vi "Chirp.vi"(0 "Pulser":T1, 1 "Agilent In":refnum<visa-resource-name>="GPIB::10::INSTR", 2 "Tabor In":refnum<k15>="Tabor2182", 3 "error in (no error)":errorcluster, 4 "Use Address?":bool=TRUE) -> (6 "error out":errorcluster)   [LabVIEW 2022 SP3]
uses:
  Pulsers/pulser.ctl
  <vilib>/Analysis/NI_AALPro.lvlib
  <vilib>/Analysis/NI_AALBase.lvlib
  Motion Controllers/-MotionRoutines/MotionGlobals.vi
  Pulsers/PulserGlobals.vi
  <vilib>/Utility/file.llb/Read From Spreadsheet File (DBL).vi
panel:
  in  "resource name":refnum<k15>
  in  "Vpp":dbl=0.105 min=0.05 max=1.0 format="%.2f"
  in  "duration tone (us)":sgl=4.0
  in  "fb (MHz)":dbl=10.0 format="%0.2f"
  in  "Tabor mode":enum32{"Arb Wave", "Sequence"}(tab)
  in  "Upload Wave?":bool
  out "Waveform Handles":i32[](array[numeric])
  in  "Clear Arb":bool
  in  "Arb Mode":bool
  in  "Arb Seg":i32=1 min=1
  in  "Scaling fac":dbl=1.0 min=-1.0 max=1.0 format="%.2f"
  in  "Clear Seq Tab":bool
  in  "Sequence Table":i32[][](array[numeric])=[[1, 1], [2, 1]] caption="Seg#      Rpt#"
  in  "Upload Seq Tab":bool
  out "seq handle":i32
  in  "dead time (us)":sgl=100.0
  in  "Tukey":dbl=0.15
  in  "Lobe ratio":dbl=90.0
  in  "duration chirp (us)":sgl=4.0
  in  "f2 (MHz)":dbl=80.0 format="%0.2f"
  in  "f1 (MHz)":dbl=10.0 format="%0.2f"
  out "Pts in Waveform":i32
  in  "Chirp File":path=path "F:/Temp/Chirp Test/Chirp12to68MHz_Tabor_9p_4us.txt"
  in  "Data Source":T2(ring)=enum."Calculate Chirp"
  in  "Func Gen":enum32{"Tabor1281", "Tabor2182", "Agilent"}(tab)=enum."Tabor2182"
  in  "T1281 D/A Rate (MHz)":dbl=1150.0 min=1.0 max=1190.0
  in  "T2182 D/A Rate (MHz)":dbl=2300.0 min=1.0 max=2300.0
  in  "User Def. Wfm Name":string="ARB_1"
  in  "samples":i32=16384
  in  "stop":bool
  out "Catalog":string
  out "Free Memory Slots":i32
  out "FFT":T3(graph)
  out "waveform":cluster{i32, dbl, dbl[]}(graph)
  # "f1 can be greater than f2. Make Tukey negative to invert chirp.\n\nUse fb for Burst and Monocycle.\n\nDuration for Chirp and Burst.\nDead time for ARFI Burst"
  # "Download before 1 Vpp change"
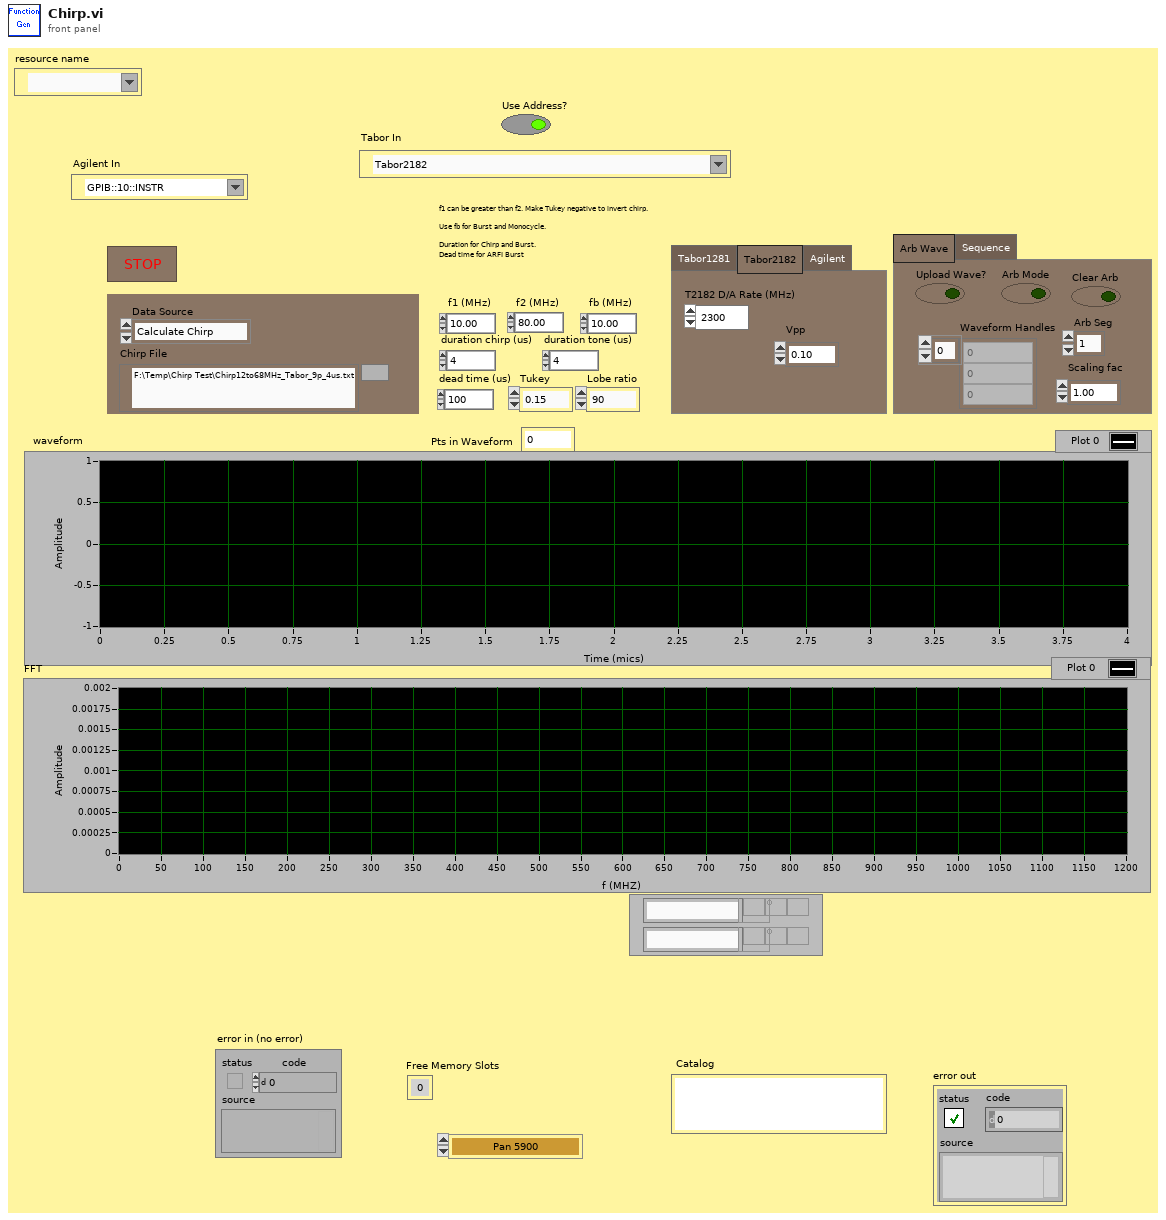
[diagram p1: front panel]
types:
  T1 = typedef "pulser.ctl" = enum16{"Pan 5900", "Daxsonics", "Agilent 33xxx", "UTEX", "JSR", "WMC Mono-Cycle", "No Pulser", "NYU AVTECH", "Tabor W1281A", "Pan 5800", "Unlisted", "Tabor WX2182B"}
  T2 = enum16{"Load Text File", "Calculate Chirp", "MonoCycle", "ToneBurst", "ARFI Burst", "ARFI Burst w/ Chirp"}
  T3 = cluster{i32, "df":dbl, "Power Spectrum (V^2 rms)":dbl[]}
  T4 = cluster{"instrument handle out":refnum<k15>, "instrument handle out":refnum<k15>, "Agilent In":refnum<visa-resource-name>}
  T5 = cluster{"Therapy frequency (MHz)":dbl, "Therapy amplitude (mV)":dbl, "time therapy on (s)":dbl, "Therapy Delay (ms) ":dbl, "Time (s)":dbl}
  T6 = cluster{"f1 (MHz)":dbl, "f2 (MHz)":dbl, "Tukey":dbl, "duration chirp (us)":sgl}
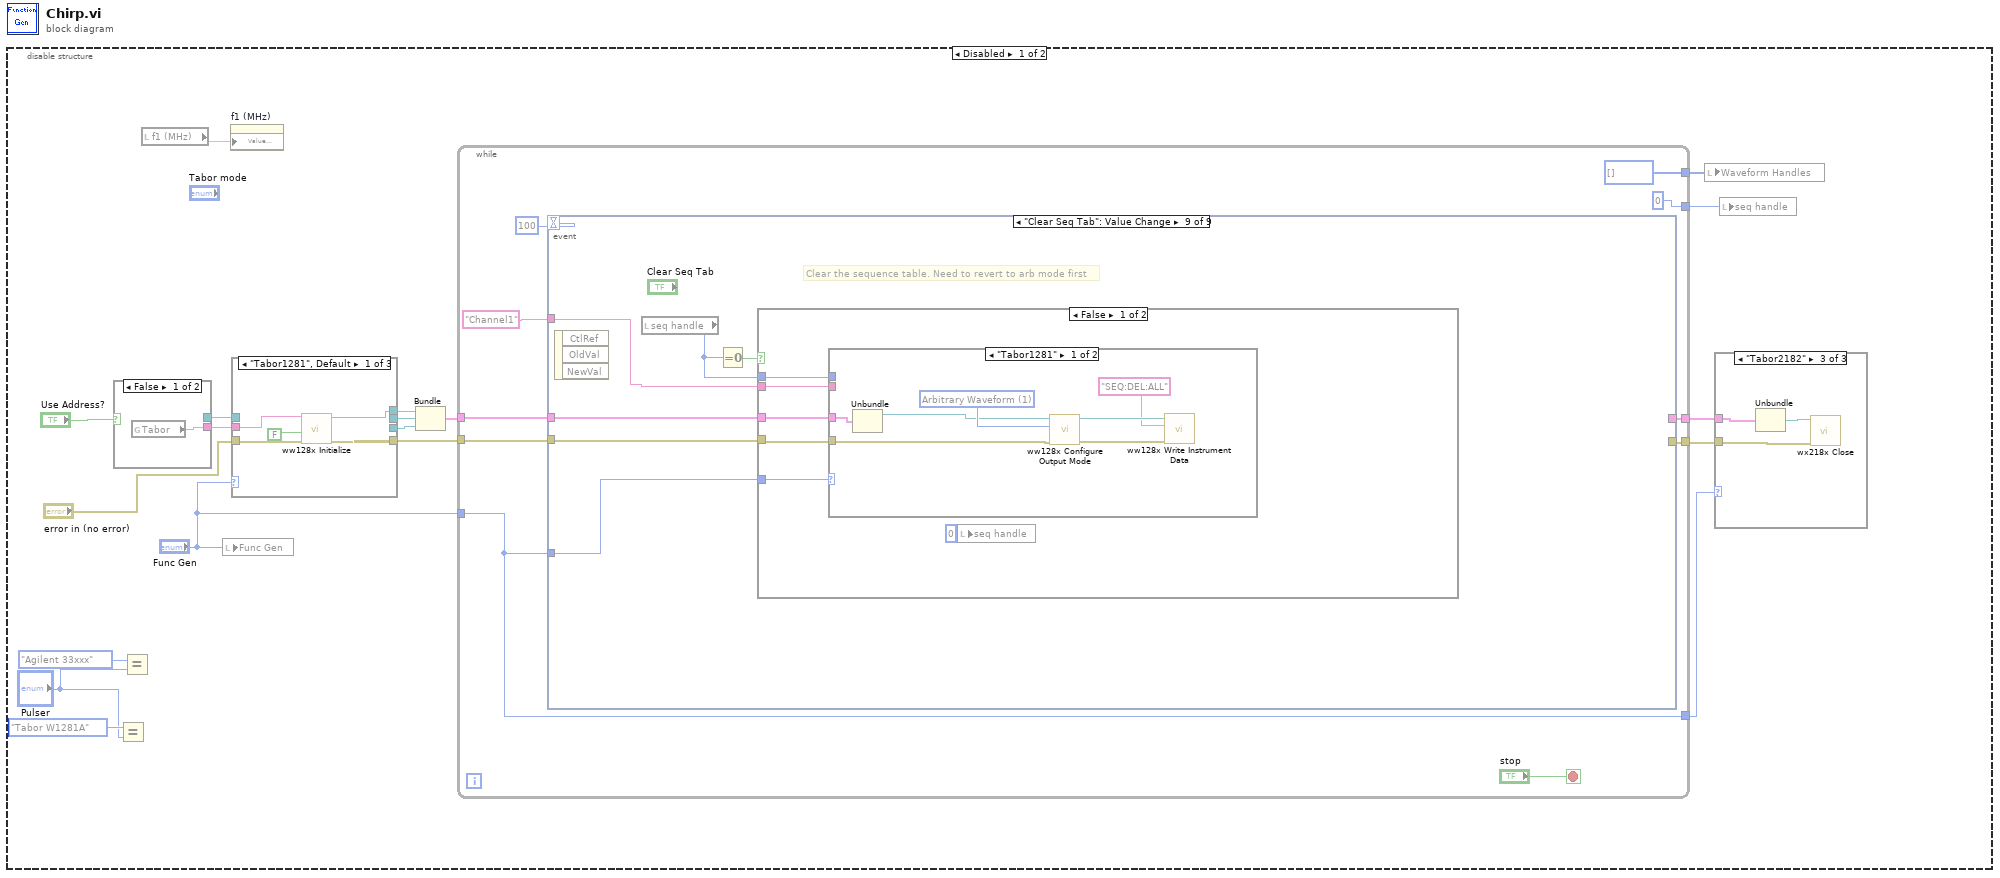
[diagram p0: block diagram]
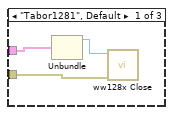
[diagram p2: hidden frame]
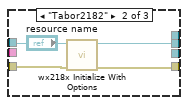
[diagram p4: hidden frame]
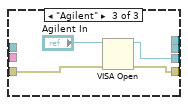
[diagram p5: hidden frame]
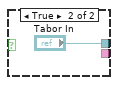
[diagram p6: hidden frame]
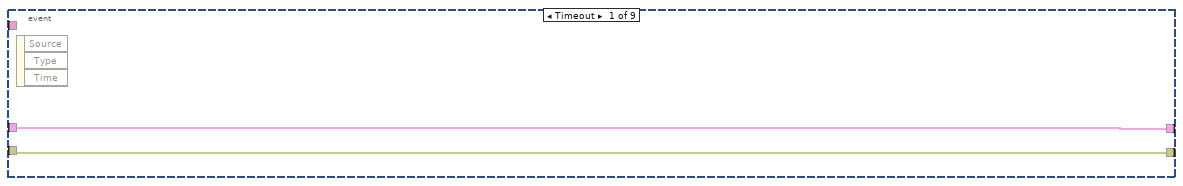
[diagram p7: hidden frame]
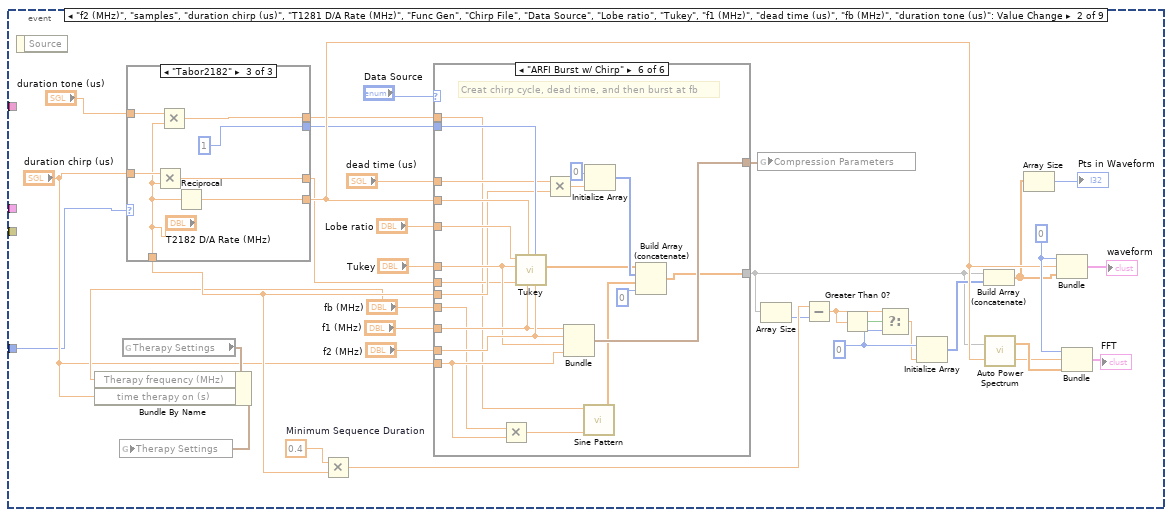
[diagram p8: hidden frame]
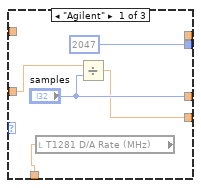
[diagram p9: hidden frame]
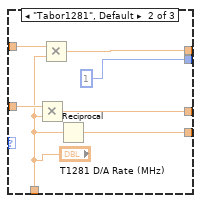
[diagram p10: hidden frame]
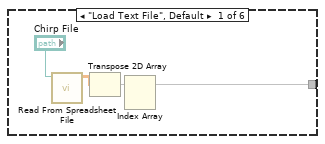
[diagram p11: hidden frame]
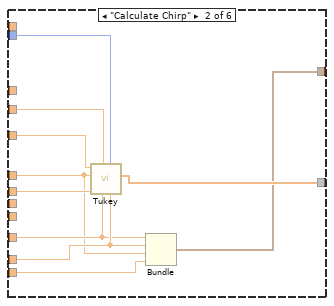
[diagram p12: hidden frame]
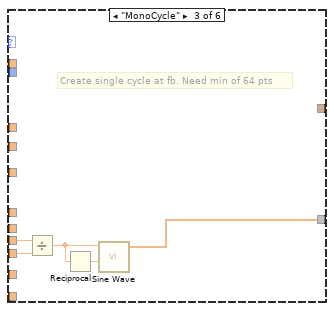
[diagram p13: hidden frame]
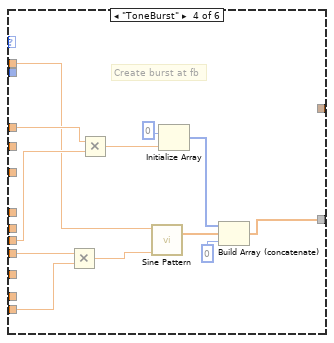
[diagram p14: hidden frame]
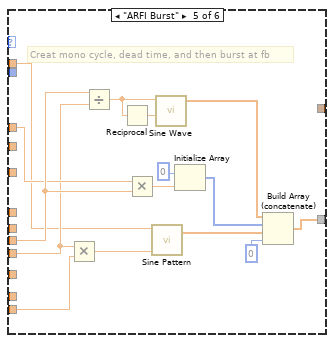
[diagram p15: hidden frame]
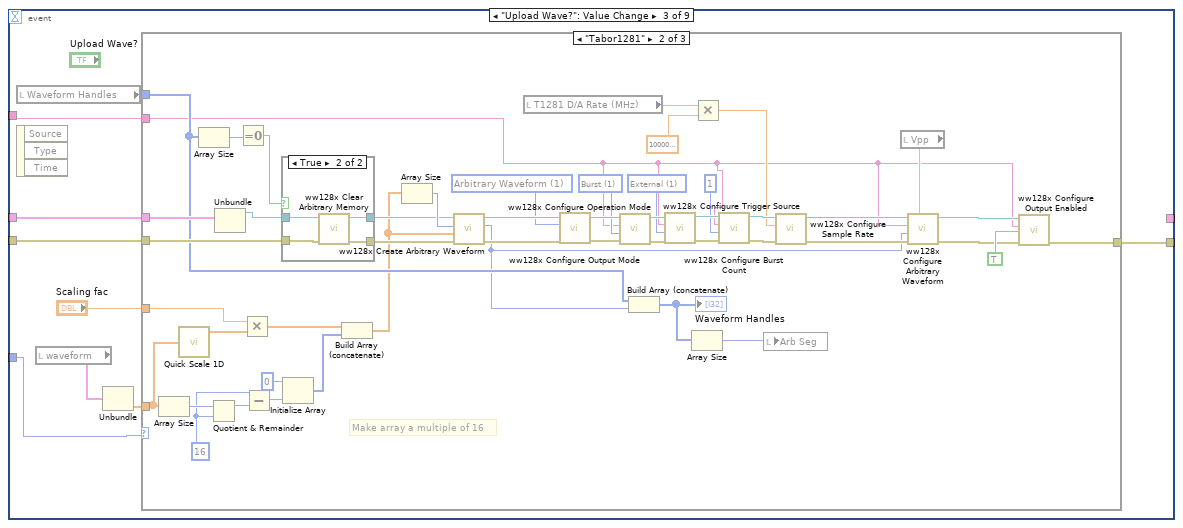
[diagram p16: hidden frame]
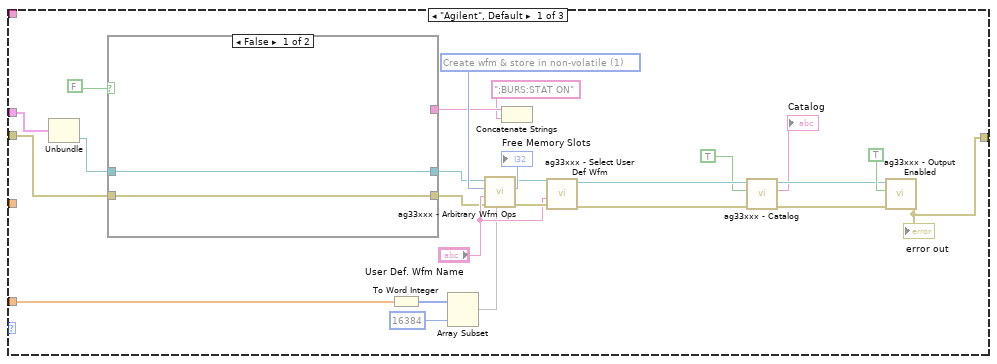
[diagram p17: hidden frame]
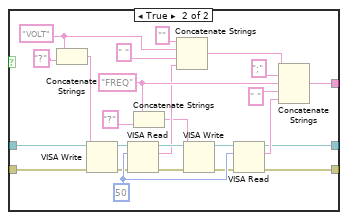
[diagram p18: hidden frame]
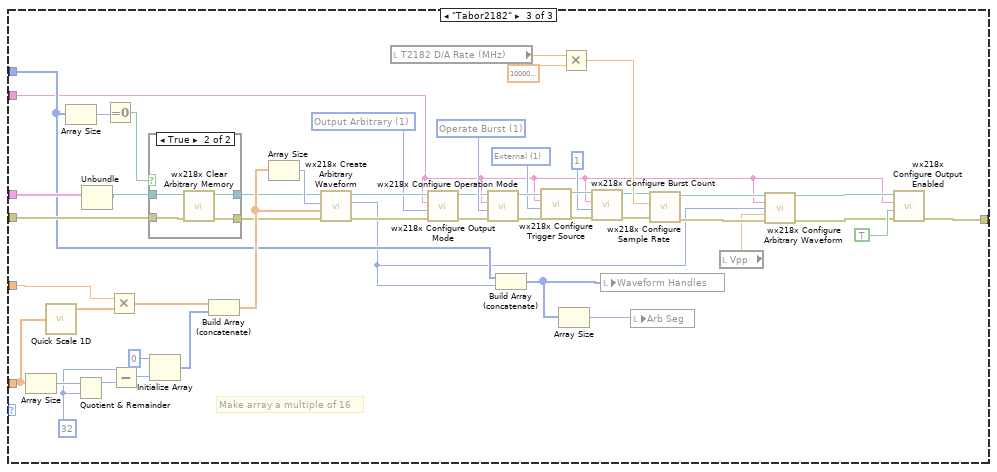
[diagram p20: hidden frame]
diagram:
  n1 = disable-structure shown="Disabled" {
    frame Disabled {
      n2 = case shown="False" "Use Address?" {
        tunnel: [w39 _] -> w2
        tunnel: [_ "Tabor In"] -> w1
        frame False {
          n3 = global read "PulserGlobals.vi" "Tabor"() -> (w39:string)
        }
        frame True {
        }
      }
      n4 = Equal?(x=pulser."Tabor W1281A", y="Pulser") -> ()  [unwired: 1 out]
      n5 = Equal?(x=pulser."Agilent 33xxx", y="Pulser") -> ()  [unwired: 1 out]
      n6 = local read "f1 (MHz)"() -> (w19:dbl)
      n7 = local write "Func Gen"("Func Gen") -> ()
      n8 = property on="f1 (MHz)" class="DigNum (strict)"("Value (Signaling)"=w19) -> ()  [unwired: 2 in, 2 out]
      n9 = case shown="\"Tabor1281\", Default" "Func Gen" {
        tunnel: [w29 w33 w36] -> w16
        tunnel: w1 -> [_ w31 _]
        tunnel: [w28 _ _] -> w12
        tunnel: [_ w34 _] -> w11
        tunnel: [_ _ w37] -> w7
        tunnel: "error in (no error)" -> [w27 w32 w35]
        tunnel: w2 -> [w26 _ _]
        frame "Tabor1281", Default {
          n10 = call <instrlib>:"ww128x Initialize.vi"("error in (no error)"=w27, "reset device (Yes)"=FALSE ("reset device"), "resource name"=w26) -> ("error out"=w29:errorcluster, "instrument handle out"=w28:refnum<k15>)  [unwired: 1 in, 6 out]
        }
        frame "Tabor2182" {
          n11 = call <instrlib>:"wx218x Initialize With Options.vi"("error in (no error)"=w32, "resource name"=w31) -> ("error out"=w33:errorcluster, "instrument handle out"=w34:refnum<k15>)  [unwired: 8 in]
        }
        frame "Agilent" {
          n12 = VISA Open(error in (no error)=w35, VISA resource name="Agilent In") -> (VISA resource name=w37:refnum<visa-resource-name>, error out=w36:errorcluster)  [unwired: 3 in]
        }
      }
      n13 = Bundle("instrument handle out"=w12, "instrument handle out"=w11, "Agilent In"=w7) -> (w10:T4)  [unwired: 1 in]
      n14 = while {
        tunnel: [w48] -> w18
        tunnel: [w47] -> w17
        tunnel: w10 -> [w46]
        tunnel: w16 -> [w45]
        tunnel: [i32[] [] ("Waveform Handles")] -> w15
        tunnel: [0 ("seq handle")] -> w13
        tunnel: "Func Gen" -> [w41]
        tunnel: [w41] -> w9
        stop <- "stop" stop-if-true
        n15 = event shown="[8] \"Clear Seq Tab\": Value Change" {
          selector: _ -> [_ _ _ _ _ _ _ _ _]
          dyn-events: _ -> [_ _ _ _ _ _ _ _ _]
          timeout: 100 -> [_ _ _ _ _ _ _ _ _]
          tunnel: [w52 _ _ _ _ _ _ _ _] -> w48
          tunnel: [w51 _ w173 _ w387 _ _ _ _] -> w47
          tunnel: w46 -> [w52 _ w179 w344 w393 w415 w469 w482 w513]
          tunnel: w45 -> [w51 _ w178 w348 w395 w416 w470 w486 w515]
          tunnel: "Channel1" -> [_ _ w175 w342 w392 w414 w467 w480 w510]
          tunnel: w41 -> [_ w53 w174 w343 w388 w413 w468 w481 w511]
          event Timeout {
            n16 = event-data() -> ()  [unwired: 4 out]
          }
          event "f2 (MHz)", "samples", "duration chirp (us)", "T1281 D/A Rate (MHz)", "Func Gen", "Chirp File", "Data Source", "Lobe ratio", "Tukey", "f1 (MHz)", "dead time (us)", "fb (MHz)", "duration tone (us)": Value Change {
            w65 = 0.4  # Minimum Sequence Duration
            w71 = 0
            w83 = 0
            n17 = event-data() -> ()  [unwired: 2 out]
            n18 = global read "PulserGlobals.vi" "Therapy Settings"() -> (w57:T5)
            n19 = Bundle By Name(cluster=w57, "Therapy frequency (MHz)"="fb (MHz)", "time therapy on (s)"="duration chirp (us)") -> (w56:T5)
            n20 = global write "PulserGlobals.vi" "Therapy Settings"(w56) -> ()
            n21 = case shown="\"Tabor2182\"" w53 {
              tunnel: ["samples" w97 w104] -> w78
              tunnel: "duration chirp (us)" -> [w91 w98 w105]
              tunnel: [w87 "T1281 D/A Rate (MHz)" "T2182 D/A Rate (MHz)"] -> w66
              tunnel: [w89 w96 w103] -> w79
              tunnel: [2047 1 1] -> w75
              tunnel: "duration tone (us)" -> [_ w94 w101]
              tunnel: [_ w93 w100] -> w58
              frame "Agilent" {
                n22 = local read "T1281 D/A Rate (MHz)"() -> (w87:dbl)
                n23 = Divide(x=w91, y="samples") -> (x/y=w89:sgl)
              }
              frame "Tabor1281", Default {
                n24 = Multiply(x=w98, y="T1281 D/A Rate (MHz)") -> (x*y=w97:dbl)
                n25 = Multiply(x=w94, y="T1281 D/A Rate (MHz)") -> (x*y=w93:dbl)
                n26 = Reciprocal(x="T1281 D/A Rate (MHz)") -> (1/x=w96:dbl)
              }
              frame "Tabor2182" {
                n27 = Multiply(x=w105, y="T2182 D/A Rate (MHz)") -> (x*y=w104:dbl)
                n28 = Multiply(x=w101, y="T2182 D/A Rate (MHz)") -> (x*y=w100:dbl)
                n29 = Reciprocal(x="T2182 D/A Rate (MHz)") -> (1/x=w103:dbl)
              }
            }
            n30 = Multiply(x=w65, y=w66) -> (x*y=w64:dbl)
            n31 = case shown="\"ARFI Burst w/ Chirp\"" "Data Source" {
              tunnel: [w107 w119 w121 w132 w147 w156] -> w67
              tunnel: "f1 (MHz)" -> [_ w115 _ _ _ w170]
              tunnel: "f2 (MHz)" -> [_ w116 _ _ _ w171]
              tunnel: w79 -> [_ w118 _ _ _ w172]
              tunnel: w78 -> [_ w117 _ _ _ w157]
              tunnel: "Lobe ratio" -> [_ w114 _ _ _ w169]
              tunnel: "Tukey" -> [_ w113 _ _ _ w168]
              tunnel: "duration chirp (us)" -> [_ w112 _ w135 w150 w154]
              tunnel: w75 -> [_ w111 _ _ _ w167]
              tunnel: w66 -> [_ _ w122 w127 w140 w158]
              tunnel: [_ w110 _ _ _ w166] -> w61
              tunnel: "dead time (us)" -> [_ _ _ w129 w139 w159]
              tunnel: "fb (MHz)" -> [_ _ w120 w126 w138 w153]
              tunnel: w58 -> [_ _ _ w125 w137 w152]
              frame "Load Text File", Default {
                n32 = call-poly <vilib>:"Read From Spreadsheet File.vi"("file path (dialog if empty)"="Chirp File") -> ("all rows"=w108:dbl[][])  [unwired: 3 in, 7 out]
                n33 = Transpose 2D Array(2D array=w108) -> (transposed array=w106:dbl[][])
                n34 = Index Array(array=w106) -> (element=w107:dbl[])  [unwired: 2 in]
              }
              frame "Calculate Chirp" {
                n35 = call "Tukey.vi"("f2 (MHz)"=w116, "Pk Value"=w111, "f1 (MHz)"=w115, "Samp Rate (mics)"=w118, "Pts"=w117, "Tukey"=w113, "Lobe ratio"=w114) -> ("Tukey Chirp"=w119:dbl[])  [unwired: 4 out]
                n36 = Bundle("f1 (MHz)"=w115, "f2 (MHz)"=w116, "Tukey"=w113, "duration chirp (us)"=w112) -> (w110:T6)  [unwired: 1 out]
              }
              frame "MonoCycle" {
                # "Create single cycle at fb. Need min of 64 pts"
                n37 = Divide(x=w122, y=w120) -> (x/y=w124:dbl)
                n38 = Reciprocal(x=w124) -> (1/x=w123:dbl)
                n39 = call <vilib>:"Sine Wave.vi"("samples"=w124, "frequency"=w123) -> ("sine wave"=w121:dbl[])  [unwired: 3 in, 2 out]
              }
              frame "ToneBurst" {
                # "Create burst at fb"
                n40 = Multiply(x=w126, y=w135) -> (x*y=w136:dbl)
                n41 = Multiply(x=w129, y=w127) -> (x*y=w130:dbl)
                n42 = call <vilib>:"Sine Pattern.vi"("cycles"=w136, "samples"=w125) -> ("Sinusoidal Pattern"=w134:dbl[])  [unwired: 2 in, 1 out]
                n43 = Initialize Array(0, w130) -> (w128:i32[])
                n44 = Build Array (concatenate)(w128, w134, 0) -> (w132:dbl[])
              }
              frame "ARFI Burst" {
                # "Creat mono cycle, dead time, and then burst at fb"
                n45 = Multiply(x=w138, y=w150) -> (x*y=w151:dbl)
                n46 = Divide(x=w140, y=w138) -> (x/y=w146:dbl)
                n47 = Reciprocal(x=w146) -> (1/x=w145:dbl)
                n48 = Multiply(x=w139, y=w140) -> (x*y=w143:dbl)
                n49 = call <vilib>:"Sine Pattern.vi"("cycles"=w151, "samples"=w137) -> ("Sinusoidal Pattern"=w149:dbl[])  [unwired: 2 in, 1 out]
                n50 = call <vilib>:"Sine Wave.vi"("samples"=w146, "frequency"=w145) -> ("sine wave"=w142:dbl[])  [unwired: 3 in, 2 out]
                n51 = Initialize Array(0, w143) -> (w141:i32[])
                n52 = Build Array (concatenate)(w142, w141, w149, 0) -> (w147:dbl[])
              }
              frame "ARFI Burst w/ Chirp" {
                # "Creat chirp cycle, dead time, and then burst at fb"
                n53 = Multiply(x=w153, y=w154) -> (x*y=w165:dbl)
                n54 = call "Tukey.vi"("f2 (MHz)"=w171, "Pk Value"=w167, "f1 (MHz)"=w170, "Samp Rate (mics)"=w172, "Pts"=w157, "Tukey"=w168, "Lobe ratio"=w169) -> ("Tukey Chirp"=w155:dbl[])  [unwired: 4 out]
                n55 = Multiply(x=w159, y=w158) -> (x*y=w161:dbl)
                n56 = Bundle("f1 (MHz)"=w170, "f2 (MHz)"=w171, "Tukey"=w168, "duration chirp (us)"=w154) -> (w166:T6)  [unwired: 1 out]
                n57 = call <vilib>:"Sine Pattern.vi"("cycles"=w165, "samples"=w152) -> ("Sinusoidal Pattern"=w164:dbl[])  [unwired: 2 in, 1 out]
                n58 = Initialize Array(0, w161) -> (w160:i32[])
                n59 = Build Array (concatenate)(w155, w160, w164, 0) -> (w156:dbl[])
              }
            }
            n60 = global write "MotionGlobals.vi" "Compression Parameters"(w61) -> ()
            n61 = Array Size(array=w67) -> (size(s)=w63:i32)
            n62 = Subtract(x=w64, y=w63) -> (x-y=w62:dbl)
            n63 = Greater Than 0?(x=w62) -> (x > 0?=w72:bool)
            n64 = Select(t=w62, s=w72, f=w71) -> (s? t:f=w70:dbl)
            n65 = Initialize Array(w71, w70) -> (w69:i32[])
            n66 = Build Array (concatenate)(w67, w69) -> (w68:dbl[])
            n67 = call <vilib>:"Auto Power Spectrum.vi"("dt"=w79, "Signal (V)"=w67) -> ("df"=w84:dbl, "Power Spectrum (V^2 rms)"=w85:dbl[])
            n68 = Array Size(array=w68) -> (size(s)=→"Pts in Waveform":i32)
            n69 = Bundle(w83, w79, w68) -> (→"waveform":cluster{i32, dbl, dbl[]})  [unwired: 1 out]
            n70 = Bundle(w83, "df"=w84, "Power Spectrum (V^2 rms)"=w85) -> (→"FFT":T3)  [unwired: 1 out]
          }
          event "Upload Wave?": Value Change {
            n71 = local read "Waveform Handles"() -> (w177:i32[])
            n72 = event-data() -> ()  [unwired: 4 out]
            n73 = local read "waveform"() -> (w181:cluster{i32, dbl, dbl[]})
            n74 = Unbundle(w181) -> (w180:dbl[])  [unwired: 2 out]
            n75 = case shown="\"Tabor1281\"" w174 {
              tunnel: w180 -> [w186 w270 w331]
              tunnel: w179 -> [w184 w247 w316]
              tunnel: w178 -> [w182 w248 w317]
              tunnel: w177 -> [_ w245 w315]
              tunnel: "Scaling fac" -> [_ w244 w314]
              tunnel: w175 -> [_ w234 w289]
              tunnel: [w185 w236 w291] -> w173
              frame "Agilent", Default {
                w206 = u16 1 items=["Create wfm & store in volatile", "Create wfm & store in non-volatile", "Copy wfm from volatile", "Delete wfm from volatile", "Delete one wfm from non-volatile", "Delete all wfms from non-volatile"] ("Mode (0: Create wfm & store in volatile)")
                n76 = Unbundle(w184) -> ("Agilent In"=w183:refnum<visa-resource-name>)  [unwired: 2 out]
                n77 = case shown="False" FALSE ("Case Constant\n(See Context Help)") {
                  tunnel: [_ w230] -> w203
                  tunnel: [w207 w212] -> w192
                  tunnel: [w208 w211] -> w191
                  tunnel: w183 -> [w207 w210]
                  tunnel: w182 -> [w208 w209]
                  frame False {
                  }
                  frame True {
                    w224 = "FREQ"
                    w227 = "VOLT"
                    w233 = u32 50
                    n78 = Concatenate Strings(w227, "?") -> (w225:string)
                    n79 = VISA Write(VISA resource name=w210, write buffer=w225, error in (no error)=w209) -> (VISA resource name out=w223:refnum<visa-resource-name>, error out=w222:errorcluster)  [unwired: 1 out]
                    n80 = VISA Read(VISA resource name=w223, byte count=w233, error in (no error)=w222) -> (VISA resource name out=w219:refnum<visa-resource-name>, read buffer=w216:string, error out=w218:errorcluster)  [unwired: 1 out]
                    n81 = Concatenate Strings(w224, "?") -> (w213:string)
                    n82 = Concatenate Strings("", w227, " ", w216) -> (w228:string)
                    n83 = VISA Write(VISA resource name=w219, write buffer=w213, error in (no error)=w218) -> (VISA resource name out=w221:refnum<visa-resource-name>, error out=w220:errorcluster)  [unwired: 1 out]
                    n84 = VISA Read(VISA resource name=w221, byte count=w233, error in (no error)=w220) -> (VISA resource name out=w212:refnum<visa-resource-name>, read buffer=w231:string, error out=w211:errorcluster)  [unwired: 1 out]
                    n85 = Concatenate Strings(w228, ";", w224, " ", w231) -> (w230:string)
                  }
                }
                n86 = To Word Integer(number=w186) -> (16bit integer=w187:i16[])
                n87 = Array Subset(array=w187, length=16384 ("samples")) -> (w189:i16[])  [unwired: 1 in]
                n88 = call <instrlib>:"ag33xxx - Arbitrary Wfm Ops.vi"("Data"=w189, "error in (no error)"=w191, "Waveform Name"="User Def. Wfm Name", "Mode (0: Create wfm & store in volatile)"=w206, "VISA session"=w192) -> ("error out"=w200:errorcluster, "Free Memory Slots"=→"Free Memory Slots":i32, "dup VISA session"=w201:refnum<visa-resource-name>)  [unwired: 4 out]
                n89 = Concatenate Strings(w203, ";BURS:STAT ON") -> ()  [unwired: 1 out]
                n90 = call <instrlib>:"ag33xxx - Select User Def Wfm.vi"("error in (no error)"=w200, "User Def. Wfm Name"="User Def. Wfm Name", "VISA session"=w201) -> ("error out"=w197:errorcluster, "dup VISA session"=w198:refnum<visa-resource-name>)  [unwired: 1 in, 6 out]
                n91 = call <instrlib>:"ag33xxx - Catalog.vi"("error in (no error)"=w197, "Location (F: User-Defined)"=TRUE, "VISA session"=w198) -> ("error out"=w196:errorcluster, "Catalog"=→"Catalog":string, "dup VISA session"=w195:refnum<visa-resource-name>)  [unwired: 6 out]
                n92 = call <instrlib>:"ag33xxx - Output Enabled.vi"("error in (no error)"=w196, "Output Enabled? (T: Yes)"=TRUE, "VISA session"=w195) -> ("error out"=w185:errorcluster)  [unwired: 8 out]
                "error out" <- w185
              }
              frame "Tabor1281" {
                w258 = 1 items=["External"=1, "Internal"=3, "Software Trigger"=2] ("source")
                w261 = 1 items=["Continuous"=0, "Burst"=1, "Gated"=1001, "Triggered"=1002] ("operation mode")
                w265 = 16
                w277 = 1 items=["Standard Function"=0, "Arbitrary Waveform"=1, "Arbitrary Sequence"=2, "Modulation"=1001] ("output mode")
                # "Make array a multiple of 16"
                n93 = Array Size(array=w270) -> (size(s)=w276:i32)
                n94 = call <vilib>:"Quick Scale 1D.vi"("X"=w270) -> ("Y[i]=X[i]/Max|X|"=w263:dbl[])  [unwired: 2 out]
                n95 = Array Size(array=w245) -> (size(s)=w252:i32)
                n96 = Quotient & Remainder(x=w276, y=w265) -> (x-y*floor(x/y)=w267:i32)  [unwired: 1 out]
                n97 = Unbundle(w247) -> ("instrument handle out"=w246:refnum<k15>)  [unwired: 2 out]
                n98 = Equal To 0?(x=w252) -> (x = 0?=w251:bool)
                n99 = Multiply(x=w244, y=w263) -> (x*y=w262:dbl[])
                n100 = Subtract(x=w265, y=w267) -> (x-y=w266:i32)
                n101 = case shown="True" w251 {
                  tunnel: w246 -> [w283 w287]
                  tunnel: [w283 w286] -> w250
                  tunnel: [w282 w285] -> w249
                  tunnel: w248 -> [w282 w284]
                  frame False {
                  }
                  frame True {
                    n102 = call <instrlib>:"ww128x Clear Arbitrary Memory.vi"("error in (no error)"=w284, "instrument handle"=w287) -> ("error out"=w285:errorcluster, "instrument handle out"=w286:refnum<k15>)  [unwired: 8 in]
                  }
                }
                n103 = Initialize Array(0, w266) -> (w274:i32[])
                n104 = Build Array (concatenate)(w262, w274) -> (w238:dbl[])
                n105 = Array Size(array=w238) -> (size(s)=w268:i32)
                n106 = call <instrlib>:"ww128x Create Arbitrary Waveform.vi"("error in (no error)"=w249, "waveform data array"=w238, "waveform size"=w268, "instrument handle"=w250) -> ("error out"=w280:errorcluster, "waveform handle"=w237:i32, "instrument handle out"=w281:refnum<k15>)  [unwired: 5 out]
                n107 = local read "T1281 D/A Rate (MHz)"() -> (w269:dbl)
                n108 = call <instrlib>:"ww128x Configure Output Mode.vi"("error in (no error)"=w280, "output mode (Standard Function)"=w277, "instrument handle"=w281) -> ("error out"=w279:errorcluster, "instrument handle out"=w278:refnum<k15>)  [unwired: 7 out]
                n109 = call <instrlib>:"ww128x Configure Operation Mode.vi"("error in (no error)"=w279, "operation mode (Continuous)"=w261, "channel name (\"CHAN_A\")"=w234, "instrument handle"=w278) -> ("error out"=w259:errorcluster, "instrument handle out"=w260:refnum<k15>)  [unwired: 6 out]
                n110 = Build Array (concatenate)(w245, w237) -> (w254:i32[])
                "Waveform Handles" <- w254
                n111 = call <instrlib>:"ww128x Configure Trigger Source.vi"("error in (no error)"=w259, "trigger source (External)"=w258, "channel name (\"CHAN_A\")"=w234, "instrument handle"=w260) -> ("error out"=w256:errorcluster, "instrument handle out"=w257:refnum<k15>)  [unwired: 6 out]
                n112 = Array Size(array=w254) -> (size(s)=w253:i32)
                n113 = Multiply(x=w269, y=1000000.0 ("sample rate")) -> (x*y=w239:dbl)
                n114 = call <instrlib>:"ww128x Configure Burst Count.vi"("error in (no error)"=w256, "burst count (2)"=1 ("burst count"), "channel name (\"CHAN_A\")"=w234, "instrument handle"=w257) -> ("error out"=w272:errorcluster, "instrument handle out"=w273:refnum<k15>)  [unwired: 6 out]
                n115 = local write "Arb Seg"(w253) -> ()
                n116 = call <instrlib>:"ww128x Configure Sample Rate.vi"("error in (no error)"=w272, "sample rate (100e6)"=w239, "instrument handle"=w273) -> ("error out"=w242:errorcluster, "instrument handle out"=w243:refnum<k15>)  [unwired: 7 out]
                n117 = local read "Vpp"() -> (w235:dbl)
                n118 = call <instrlib>:"ww128x Configure Arbitrary Waveform.vi"("gain (1.00)"=w235, "error in (no error)"=w242, "waveform handle (10000)"=w237, "channel name (\"CHAN_A\")"=w234, "instrument handle"=w243) -> ("error out"=w241:errorcluster, "instrument handle out"=w240:refnum<k15>)  [unwired: 5 in]
                n119 = call <instrlib>:"ww128x Configure Output Enabled.vi"("error in (no error)"=w241, "channel enabled (False)"=TRUE ("output enable"), "channel name (\"CHAN_A\")"=w234, "instrument handle"=w240) -> ("error out"=w236:errorcluster)  [unwired: 7 out]
              }
              frame "Tabor2182" {
                w290 = 1 items=["Output Function", "Output Arbitrary", "Output Sequence"] ("output mode (Output Function)")
                w308 = 1 items=["External"=1, "Software Trigger"=2, "Internal Trigger"=3, "TTL0"=111, "TTL1"=112, "TTL2"=113, "TTL3"=114, "TTL4"=115, "TTL5"=116, "TTL6"=117, "TTL7"=118, "ECL0"=119, "ECL1"=120, "PXI Star"=131, "RTSI0"=141, "RTSI1"=142, "RTSI2"=143, "RTSI3"=144, "RTSI4"=145, "RTSI5"=146, "RTSI6"=147] ("trigger source (External)")
                w311 = 1 items=["Operate Continuous", "Operate Burst"] ("operation mode (Operate Continuous)")
                w325 = 32
                # "Make array a multiple of 16"
                n120 = Array Size(array=w331) -> (size(s)=w335:i32)
                n121 = call <vilib>:"Quick Scale 1D.vi"("X"=w331) -> ("Y[i]=X[i]/Max|X|"=w324:dbl[])  [unwired: 2 out]
                n122 = Array Size(array=w315) -> (size(s)=w321:i32)
                n123 = Quotient & Remainder(x=w335, y=w325) -> (x-y*floor(x/y)=w327:i32)  [unwired: 1 out]
                n124 = Unbundle(w316) -> ("instrument handle out"=w312:refnum<k15>)  [unwired: 2 out]
                n125 = Equal To 0?(x=w321) -> (x = 0?=w320:bool)
                n126 = Multiply(x=w314, y=w324) -> (x*y=w323:dbl[])
                n127 = Subtract(x=w325, y=w327) -> (x-y=w326:i32)
                n128 = case shown="True" w320 {
                  tunnel: w312 -> [w337 w338]
                  tunnel: [w337 w341] -> w319
                  tunnel: [w336 w340] -> w318
                  tunnel: w317 -> [w336 w339]
                  frame False {
                  }
                  frame True {
                    n129 = call <instrlib>:"wx218x Clear Arbitrary Memory.vi"("error in (no error)"=w339, "instrument handle"=w338) -> ("error out"=w340:errorcluster, "instrument handle out"=w341:refnum<k15>)  [unwired: 8 in]
                  }
                }
                n130 = Initialize Array(0, w326) -> (w333:i32[])
                n131 = Build Array (concatenate)(w323, w333) -> (w329:dbl[])
                n132 = Array Size(array=w329) -> (size(s)=w328:i32)
                n133 = call <instrlib>:"wx218x Create Arbitrary Waveform.vi"("error in (no error)"=w318, "Waveform Data Array (empty)"=w329, "Waveform Size (0)"=w328, "instrument handle"=w319) -> ("error out"=w298:errorcluster, "Waveform Handle"=w292:i32, "instrument handle out"=w301:refnum<k15>)  [unwired: 5 in]
                n134 = local read "T2182 D/A Rate (MHz)"() -> (w330:dbl)
                n135 = call <instrlib>:"wx218x Configure Output Mode.vi"("error in (no error)"=w298, "OutputMode (Output Mode Function)"=w290, "Channel"=w289, "instrument handle"=w301) -> ("error out"=w299:errorcluster, "instrument handle out"=w300:refnum<k15>)  [unwired: 6 in]
                n136 = call <instrlib>:"wx218x Configure Operation Mode.vi"("error in (no error)"=w299, "OperationMode (Operation Mode Continuous)"=w311, "Channel"=w289, "instrument handle"=w300) -> ("error out"=w309:errorcluster, "instrument handle out"=w310:refnum<k15>)  [unwired: 6 in]
                n137 = Build Array (concatenate)(w315, w292) -> (w313:i32[])
                n138 = call <instrlib>:"wx218x Configure Trigger Source.vi"("error in (no error)"=w309, "Source (Trigger Source External)"=w308, "Channel"=w289, "instrument handle"=w310) -> ("error out"=w306:errorcluster, "instrument handle out"=w307:refnum<k15>)  [unwired: 6 in]
                n139 = Array Size(array=w313) -> (size(s)=w322:i32)
                n140 = Multiply(x=w330, y=1000000.0 ("sample rate")) -> (x*y=w304:dbl)
                n141 = call <instrlib>:"wx218x Configure Burst Count.vi"("error in (no error)"=w306, "Count"=1 ("burst count"), "Channel"=w289, "instrument handle"=w307) -> ("error out"=w302:errorcluster, "instrument handle out"=w303:refnum<k15>)  [unwired: 6 in]
                n142 = local write "Waveform Handles"(w313) -> ()
                n143 = local write "Arb Seg"(w322) -> ()
                n144 = call <instrlib>:"wx218x Configure Sample Rate.vi"("error in (no error)"=w302, "SampleRate"=w304, "instrument handle"=w303) -> ("error out"=w293:errorcluster, "instrument handle out"=w296:refnum<k15>)  [unwired: 7 in]
                n145 = local read "Vpp"() -> (w288:dbl)
                n146 = call <instrlib>:"wx218x Configure Arbitrary Waveform.vi"("instrument handle"=w296, "Channel Name (\"CHANNEL1\")"=w289, "Waveform Handle (0)"=w292, "Gain (1.00)"=w288, "error in (no error)"=w293) -> ("instrument handle out"=w295:refnum<k15>, "error out"=w294:errorcluster)  [unwired: 9 in]
                n147 = call <instrlib>:"wx218x Configure Output Enabled.vi"("error in (no error)"=w294, "Channel Enabled (Off)"=TRUE ("output enable"), "Channel Name"=w289, "instrument handle"=w295) -> ("error out"=w291:errorcluster)  [unwired: 6 in, 1 out]
              }
            }
          }
          event "Clear Arb": Value Change {
            # "Clear All Arb Waves"
            n148 = event-data() -> ()  [unwired: 3 out]
            n149 = local read "Waveform Handles"() -> (w347:i32[])
            n150 = Array Size(array=w347) -> (size(s)=w345:i32)
            n151 = Not Equal To 0?(x=w345) -> (x != 0?=w346:bool)
            n152 = case shown="\"Tabor1281\", Default" w343 {
              tunnel: w348 -> [w359 w379]
              tunnel: w346 -> [w351 w375]
              tunnel: w344 -> [w350 w381]
              tunnel: w342 -> [_ w372]
              frame "Tabor1281", Default {
                w358 = 0 items=["Standard Function", "Arbitrary Waveform", "Arbitrary Sequence"] ("output mode")
                n153 = Unbundle(w350) -> ("instrument handle out"=w349:refnum<k15>)  [unwired: 2 out]
                n154 = local read "seq handle"() -> (w355:i32)
                n155 = call <instrlib>:"ww128x Configure Output Mode.vi"("error in (no error)"=w359, "output mode (Standard Function)"=w358, "instrument handle"=w349) -> ("error out"=w356:errorcluster, "instrument handle out"=w357:refnum<k15>)  [unwired: 7 out]
                n156 = Equal To 0?(x=w355) -> (x = 0?=w354:bool)
                n157 = case shown="False" w354 {
                  tunnel: w357 -> [w368 w371]
                  tunnel: w356 -> [w367 w370]
                  tunnel: [w366 w371] -> w353
                  tunnel: [w365 w370] -> w352
                  frame False {
                    n158 = local write "seq handle"(0 ("seq handle")) -> ()
                    n159 = call <instrlib>:"ww128x Write Instrument Data.vi"("error in (no error)"=w367, "write buffer"="SEQ:DEL:ALL", "instrument handle"=w368) -> ("error out"=w365:errorcluster, "instrument handle out"=w366:refnum<k15>)  [unwired: 7 out]
                  }
                  frame True {
                  }
                }
                n160 = case shown="True" w351 {
                  tunnel: w353 -> [_ w362]
                  tunnel: w352 -> [_ w361]
                  frame False {
                  }
                  frame True {
                    n161 = local write "Waveform Handles"(i32[] [] ("Waveform Handles")) -> ()
                    n162 = call <instrlib>:"ww128x Write Instrument Data.vi"("error in (no error)"=w361, "write buffer"="TRAC:DEL:ALL", "instrument handle"=w362) -> ()  [unwired: 9 out]
                  }
                }
              }
              frame "Tabor2182" {
                w373 = 0 items=["Output Function", "Output Arbitrary", "Output Sequence"] ("output mode (Output Function)")
                n163 = Unbundle(w381) -> ("instrument handle out"=w380:refnum<k15>)  [unwired: 2 out]
                n164 = call <instrlib>:"wx218x Configure Output Mode.vi"("error in (no error)"=w379, "OutputMode (Output Mode Function)"=w373, "Channel"=w372, "instrument handle"=w380) -> ("error out"=w377:errorcluster, "instrument handle out"=w378:refnum<k15>)  [unwired: 6 in]
                n165 = local read "seq handle"() -> (w382:i32)
                n166 = Not Equal To 0?(x=w382) -> (x != 0?=w376:bool)
                n167 = Or(x=w375, y=w376) -> (x .or. y?=w374:bool)
                n168 = case shown="True" w374 {
                  tunnel: w378 -> [_ w385]
                  tunnel: w377 -> [_ w384]
                  frame False {
                  }
                  frame True {
                    n169 = call <instrlib>:"wx218x Clear Arbitrary Memory.vi"("error in (no error)"=w384, "instrument handle"=w385) -> ()  [unwired: 8 in, 2 out]
                    n170 = local write "Waveform Handles"(i32[] [] ("Waveform Handles")) -> ()
                    n171 = local write "seq handle"(0 ("seq handle")) -> ()
                  }
                }
              }
            }
          }
          event "Vpp": Value Change {
            # "Set Vpp"
            n172 = event-data() -> ("NewVal"=w394:dbl)  [unwired: 2 out]
            n173 = case shown="\"Tabor2182\"" w388 {
              tunnel: w395 -> [w404 w409]
              tunnel: w394 -> [w400 w405]
              tunnel: w393 -> [w399 w412]
              tunnel: w392 -> [_ w410]
              tunnel: [w397 w406] -> w387
              frame "Tabor1281", Default {
                n174 = Unbundle(w399) -> ("instrument handle out"=w398:refnum<k15>)  [unwired: 2 out]
                n175 = Number To Exponential String(number=w400) -> (E-format string=w402:string)  [unwired: 3 out]
                n176 = Concatenate Strings("VOLT" ("string"), w402) -> (w403:string)
                n177 = call <instrlib>:"ww128x Write Instrument Data.vi"("error in (no error)"=w404, "write buffer"=w403, "instrument handle"=w398) -> ("error out"=w397:errorcluster)  [unwired: 8 out]
              }
              frame "Tabor2182" {
                n178 = local read "Waveform Handles"() -> (w408:i32[])
                n179 = Unbundle(w412) -> ("instrument handle out"=w411:refnum<k15>)  [unwired: 2 out]
                n180 = Index Array(array=w408) -> (element=w407:i32)  [unwired: 1 in]
                n181 = call <instrlib>:"wx218x Configure Arbitrary Waveform.vi"("instrument handle"=w411, "Channel Name (\"CHANNEL1\")"=w410, "Waveform Handle (0)"=w407, "Gain (1.00)"=w405, "error in (no error)"=w409) -> ("error out"=w406:errorcluster)  [unwired: 9 in, 1 out]
              }
            }
            n182 = Multiply(x=w394, y=1000) -> (x*y=w389:dbl)
            n183 = global read "PulserGlobals.vi" "Therapy Settings"() -> (w391:T5)
            n184 = Bundle By Name(cluster=w391, "Therapy amplitude (mV)"=w389) -> (w390:T5)
            n185 = global write "PulserGlobals.vi" "Therapy Settings"(w390) -> ()
          }
          event "Upload Seq Tab": Value Change {
            # "Upload the sequence table. Waveform and number of repeats"
            # "Configure for sequence mode."
            n186 = event-data() -> ()  [unwired: 3 out]
            n187 = local read "Waveform Handles"() -> (w421:i32[])
            n188 = Index Array(array="Sequence Table", index (col)=0 ("disabled index (col)")) -> (element=w423:i32[])  [unwired: 1 in]
            n189 = Index Array(array="Sequence Table", index (col)=1 ("disabled index (col)")) -> (element=w419:i32[])  [unwired: 1 in]
            n190 = Decrement(x=w423) -> (x-1=w422:i32[])
            n191 = for {
              tunnel: w422 -> [w465] mode=indexing
              tunnel: w421 -> [w466]
              tunnel: [w464] -> w420 mode=indexing
              n192 = Index Array(array=w466, index=w465) -> (element=w464:i32)
            }
            n193 = Array Size(array=w419) -> (size(s)=w418:i32)
            n194 = case shown="\"Tabor2182\"" w413 {
              tunnel: w420 -> [w428 _ w449]
              tunnel: w419 -> [w429 _ w459]
              tunnel: w418 -> [w436 _ w458]
              tunnel: [w435 _ w457] -> w417
              tunnel: w416 -> [w434 _ w461]
              tunnel: w415 -> [w431 _ w463]
              tunnel: w414 -> [w427 _ w447]
              frame "Tabor1281", Default {
                w439 = 1002 items=["Continuous"=0, "Burst"=1, "Gated"=1001, "Triggered"=1002] ("operation mode")
                w440 = 3 items=["Auto", "Step", "Single", "RSingle", "Mix"] ("sequence advance")
                w445 = 2 items=["Standard Function", "Arbitrary Waveform", "Arbitrary Sequence"] ("output mode")
                n195 = Unbundle(w431) -> ("instrument handle out"=w430:refnum<k15>)  [unwired: 2 out]
                n196 = call <instrlib>:"ww128x Configure Operation Mode.vi"("error in (no error)"=w434, "operation mode (Continuous)"=w439, "channel name (\"CHAN_A\")"=w427, "instrument handle"=w430) -> ("error out"=w437:errorcluster, "instrument handle out"=w438:refnum<k15>)  [unwired: 6 out]
                n197 = call <instrlib>:"ww128x Create Arbitrary Sequence.vi"("loop counts array"=w429, "waveform handles array"=w428, "error in (no error)"=w437, "sequence length"=w436, "instrument handle"=w438) -> ("error out"=w432:errorcluster, "sequence handle"=w435:i32, "instrument handle out"=w433:refnum<k15>)  [unwired: 4 out]
                n198 = call <instrlib>:"ww128x Configure Sequence Advance.vi"("error in (no error)"=w432, "Sequence Advance (Auto)"=w440, "instrument handle"=w433) -> ("error out"=w441:errorcluster, "instrument handle out"=w442:refnum<k15>)  [unwired: 1 in, 6 out]
                n199 = call <instrlib>:"ww128x Configure Output Enabled.vi"("error in (no error)"=w441, "channel enabled (False)"=TRUE ("output enable"), "channel name (\"CHAN_A\")"=w427, "instrument handle"=w442) -> ("error out"=w443:errorcluster, "instrument handle out"=w444:refnum<k15>)  [unwired: 6 out]
                n200 = call <instrlib>:"ww128x Configure Output Mode.vi"("error in (no error)"=w443, "output mode (Standard Function)"=w445, "instrument handle"=w444) -> ()  [unwired: 9 out]
              }
              frame "Agilent" {
              }
              frame "Tabor2182" {
                w448 = 2 items=["Output Function", "Output Arbitrary", "Output Sequence"] ("output mode (Output Function)")
                w460 = 1 items=["Operate Continuous", "Operate Burst"] ("operation mode (Operate Continuous)")
                n201 = Unbundle(w463) -> ("instrument handle out"=w462:refnum<k15>)  [unwired: 2 out]
                n202 = call <instrlib>:"wx218x Configure Operation Mode.vi"("error in (no error)"=w461, "OperationMode (Operation Mode Continuous)"=w460, "Channel"=w447, "instrument handle"=w462) -> ("error out"=w456:errorcluster, "instrument handle out"=w455:refnum<k15>)  [unwired: 6 in]
                n203 = call <instrlib>:"wx218x Create Arbitrary Sequence.vi"("instrument handle"=w455, "WfmHandleBufferSize"=w458, "Waveform Handles Array (empty)"=w449, "Loop Counts Array (empty)"=w459, "error in (no error)"=w456) -> ("instrument handle out"=w451:refnum<k15>, "Sequence Handle"=w457:i32, "error out"=w450:errorcluster)  [unwired: 8 in]
                n204 = call <instrlib>:"wx218x Configure Output Enabled.vi"("error in (no error)"=w450, "Channel Enabled (Off)"=TRUE ("output enable"), "Channel Name"=w447, "instrument handle"=w451) -> ("error out"=w452:errorcluster, "instrument handle out"=w453:refnum<k15>)  [unwired: 6 in]
                n205 = call <instrlib>:"wx218x Configure Output Mode.vi"("error in (no error)"=w452, "OutputMode (Output Mode Function)"=w448, "Channel"=w447, "instrument handle"=w453) -> ()  [unwired: 6 in, 2 out]
              }
            }
            "seq handle" <- w417
          }
          event "Arb Mode": Value Change {
            # "Place back in Arb mode"
            n206 = event-data() -> ()  [unwired: 5 out]
            n207 = case shown="\"Tabor2182\"" w468 {
              tunnel: w470 -> [w473 w477]
              tunnel: w469 -> [w472 w479]
              tunnel: w467 -> [_ w475]
              frame "Tabor1281", Default {
                w474 = 1 items=["Standard Function", "Arbitrary Waveform", "Arbitrary Sequence"] ("output mode")
                n208 = Unbundle(w472) -> ("instrument handle out"=w471:refnum<k15>)  [unwired: 2 out]
                n209 = call <instrlib>:"ww128x Configure Output Mode.vi"("error in (no error)"=w473, "output mode (Standard Function)"=w474, "instrument handle"=w471) -> ()  [unwired: 9 out]
              }
              frame "Tabor2182" {
                w476 = 1 items=["Output Function", "Output Arbitrary", "Output Sequence"] ("output mode (Output Function)")
                n210 = Unbundle(w479) -> ("instrument handle out"=w478:refnum<k15>)  [unwired: 2 out]
                n211 = call <instrlib>:"wx218x Configure Output Mode.vi"("error in (no error)"=w477, "OutputMode (Output Mode Function)"=w476, "Channel"=w475, "instrument handle"=w478) -> ()  [unwired: 6 in, 2 out]
              }
            }
          }
          event "Arb Seg": Value Change {
            # "Choose the Arb seg to see. Index starts at 1"
            n212 = event-data() -> ("NewVal"=w487:i32)  [unwired: 3 out]
            n213 = local read "Waveform Handles"() -> (w483:i32[])
            n214 = Array Size(array=w483) -> (size(s)=w484:i32)
            n215 = Equal To 0?(x=w484) -> (x = 0?=w485:bool)
            n216 = case shown="False" w485 {
              tunnel: w487 -> [w491 _]
              tunnel: w486 -> [w492 _]
              tunnel: w482 -> [w490 _]
              tunnel: w481 -> [w489 _]
              tunnel: w480 -> [w488 _]
              frame False {
                n217 = case shown="\"Tabor1281\", Default" w489 {
                  tunnel: w492 -> [w501 w507]
                  tunnel: w491 -> [w498 _]
                  tunnel: w490 -> [w494 w508]
                  tunnel: w488 -> [_ w503]
                  frame "Tabor1281", Default {
                    w502 = 1 items=["Standard Function", "Arbitrary Waveform", "Arbitrary Sequence"] ("output mode")
                    n218 = Unbundle(w494) -> ("instrument handle out"=w493:refnum<k15>)  [unwired: 2 out]
                    n219 = call <instrlib>:"ww128x Configure Output Mode.vi"("error in (no error)"=w501, "output mode (Standard Function)"=w502, "instrument handle"=w493) -> ("error out"=w495:errorcluster, "instrument handle out"=w496:refnum<k15>)  [unwired: 7 out]
                    n220 = Number To Decimal String(number=w498) -> (decimal integer string=w497:string)  [unwired: 1 in]
                    n221 = Concatenate Strings("TRAC:SEL" ("string"), w497) -> (w499:string)
                    n222 = call <instrlib>:"ww128x Write Instrument Data.vi"("error in (no error)"=w495, "write buffer"=w499, "instrument handle"=w496) -> ()  [unwired: 9 out]
                  }
                  frame "Tabor2182" {
                    w504 = 1 items=["Output Function", "Output Arbitrary", "Output Sequence"] ("output mode (Output Function)")
                    n223 = Unbundle(w508) -> ("instrument handle out"=w509:refnum<k15>)  [unwired: 2 out]
                    n224 = call <instrlib>:"wx218x Configure Output Mode.vi"("error in (no error)"=w507, "OutputMode (Output Mode Function)"=w504, "Channel"=w503, "instrument handle"=w509) -> ("error out"=w505:errorcluster, "instrument handle out"=w506:refnum<k15>)  [unwired: 6 in]
                    n225 = call <instrlib>:"wx218x Clear Memory.vi"("error in (no error)"=w505, "instrument handle"=w506) -> ()  [unwired: 8 in, 2 out]
                  }
                }
              }
              frame True {
              }
            }
          }
          event "Clear Seq Tab": Value Change {
            # "Clear the sequence table. Need to revert to arb mode first"
            n226 = event-data() -> ()  [unwired: 4 out]
            n227 = local read "seq handle"() -> (w512:i32)
            n228 = Equal To 0?(x=w512) -> (x = 0?=w514:bool)
            n229 = case shown="False" w514 {
              tunnel: w515 -> [w521 _]
              tunnel: w513 -> [w519 _]
              tunnel: w511 -> [w518 _]
              tunnel: w512 -> [w517 _]
              tunnel: w510 -> [w516 _]
              frame False {
                n230 = case shown="\"Tabor1281\"" w518 {
                  tunnel: w521 -> [w527 w534]
                  tunnel: w519 -> [w523 w535]
                  tunnel: w517 -> [_ w529]
                  tunnel: w516 -> [_ w530]
                  frame "Tabor1281" {
                    w528 = 1 items=["Standard Function", "Arbitrary Waveform", "Arbitrary Sequence"] ("output mode")
                    n231 = Unbundle(w523) -> ("instrument handle out"=w522:refnum<k15>)  [unwired: 2 out]
                    n232 = call <instrlib>:"ww128x Configure Output Mode.vi"("error in (no error)"=w527, "output mode (Standard Function)"=w528, "instrument handle"=w522) -> ("error out"=w525:errorcluster, "instrument handle out"=w526:refnum<k15>)  [unwired: 7 out]
                    n233 = call <instrlib>:"ww128x Write Instrument Data.vi"("error in (no error)"=w525, "write buffer"="SEQ:DEL:ALL", "instrument handle"=w526) -> ()  [unwired: 9 out]
                  }
                  frame "Tabor2182", Default {
                    w531 = 1 items=["Output Function", "Output Arbitrary", "Output Sequence"] ("output mode (Output Function)")
                    n234 = Unbundle(w535) -> ("instrument handle out"=w536:refnum<k15>)  [unwired: 2 out]
                    n235 = call <instrlib>:"wx218x Configure Output Mode.vi"("error in (no error)"=w534, "OutputMode (Output Mode Function)"=w531, "Channel"=w530, "instrument handle"=w536) -> ("error out"=w532:errorcluster, "instrument handle out"=w533:refnum<k15>)  [unwired: 6 in]
                    n236 = call <instrlib>:"wx218x Clear Arbitrary Sequence.vi"("error in (no error)"=w532, "Sequence Handle (0)"=w529, "instrument handle"=w533) -> ()  [unwired: 7 in, 2 out]
                  }
                }
                n237 = local write "seq handle"(0 ("seq handle")) -> ()
              }
              frame True {
              }
            }
          }
        }
      }
      n238 = local write "Waveform Handles"(w15) -> ()
      n239 = case shown="\"Tabor2182\"" w9 {
        tunnel: w18 -> [w21 _ w24]
        tunnel: w17 -> [w22 _ w25]
        frame "Tabor1281", Default {
          n240 = Unbundle(w21) -> ("instrument handle out"=w20:refnum<k15>)  [unwired: 2 out]
          n241 = call <instrlib>:"ww128x Close.vi"("error in (no error)"=w22, "instrument handle"=w20) -> ()  [unwired: 10 out]
        }
        frame "Agilent" {
        }
        frame "Tabor2182" {
          n242 = Unbundle(w24) -> ("instrument handle out"=w23:refnum<k15>)  [unwired: 2 out]
          n243 = call <instrlib>:"wx218x Close.vi"("error in (no error)"=w25, "instrument handle"=w23) -> ()  [unwired: 9 in, 1 out]
        }
      }
      n244 = local write "seq handle"(w13) -> ()
    }
    frame Enabled {
    }
  }
